vi "DriveModeController.vi"(0 "Selected State (In)":string) -> (1 "Drive Mode Change":bool, 2 "Drive Mode":T1(ring))   [LabVIEW 2019]
doc: "This VI manages the robot drive mode. The default mode is driver control in which the swerve drive accepts all drive inputs and seemlessly combines them with autonomous corrections. Two auto targeting modes are also implimented."
uses:
  dsinstructions.vi
  sensors.vi
  dsdata.vi
  outputs.vi
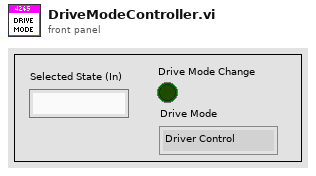
[diagram p1: front panel]
types:
  T1 = enum16{"Driver Control", "Auto Targeting", "Feeder Station"}
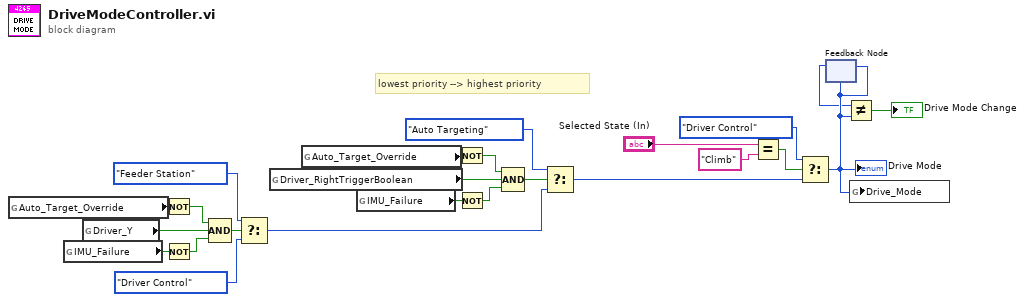
[diagram p0: block diagram]
diagram:
  # "lowest priority --> highest priority"
  n1 = global read "dsdata.vi" "Auto_Target_Override"() -> (w9:bool)
  n2 = global read "sensors.vi" "IMU_Failure"() -> (w7:bool)
  n3 = global read "dsinstructions.vi" "Driver_Y"() -> (w10:bool)
  n4 = Not(x=w9) -> (.not. x?=w8:bool)
  n5 = Not(x=w7) -> (.not. x?=w6:bool)
  n6 = Compound Arithmetic op=AND(w8, w10, w6) -> (w5:bool)
  n7 = Select(t=T1."Feeder Station", s=w5, f=T1."Driver Control") -> (s? t:f=w23:T1)
  n8 = global read "dsinstructions.vi" "Driver_RightTriggerBoolean"() -> (w20:bool)
  n9 = global read "dsdata.vi" "Auto_Target_Override"() -> (w16:bool)
  n10 = global read "sensors.vi" "IMU_Failure"() -> (w14:bool)
  n11 = Not(x=w16) -> (.not. x?=w15:bool)
  n12 = Not(x=w14) -> (.not. x?=w13:bool)
  n13 = Compound Arithmetic op=AND(w15, w20, w13) -> (w4:bool)
  n14 = Select(t=T1."Auto Targeting", s=w4, f=w23) -> (s? t:f=w24:T1)
  n15 = Equal?(x="Selected State (In)", y="Climb") -> (x = y?=w19:bool)
  n16 = Select(t=T1."Driver Control", s=w19, f=w24) -> (s? t:f=w3:T1)
  "Drive Mode" <- w3
  n17 = feedback #1(w3) -> (w2:T1)
  n18 = feedback-in #1(w3) -> ()
  n19 = Not Equal?(x=w2, y=w3) -> (x != y?=→"Drive Mode Change":bool)
  n20 = global write "outputs.vi" "Drive_Mode"(w3) -> ()
